vi "Lock VIs.vi"() -> ()   [LabVIEW 2017]
uses:
  KATE/Files/File Utils.lvlib
panel:
  out "Busy":bool
  in  "Reset":bool
  in  "Files":T1(array[cluster]) caption="Folder                                                                                Name                                   Protect"
  in  "Unlock":bool
  in  "Lock":bool
  in  "Get Files":bool
  out "Unlocked Cnt":i32
  out "Locked Cnt":i32
  in  "Lock PW":string="KwestEng#8002"
  in  "Unlock PW":string
  in  "Folder":path
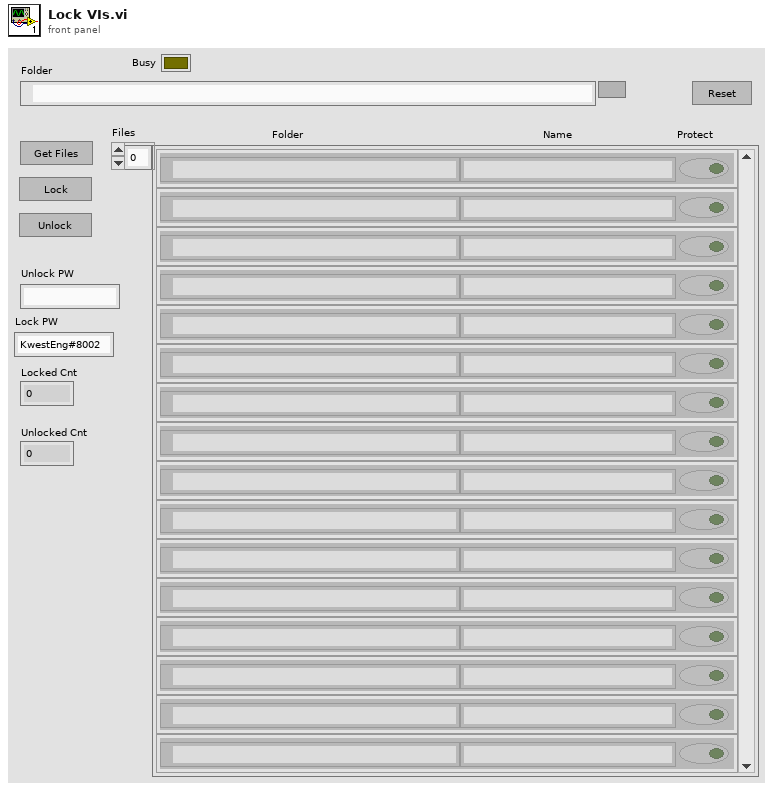
[diagram p1: front panel]
types:
  T1 = cluster{"Name":string, "Folder":path, "Protected":bool}[]
  T2 = cluster{"Name":string, "Folder":path, "Protected":bool}
  T3 = enum32{"invalid lock state", "Not Locked", "Locked (No Password)", "Password-protected"}
  T4 = cluster{"Files":cluster{"Name":string, "Folder":path, "Protected":bool}[], "UnlockPW":string, "LockPW":string}
  T5 = enum8{"Enabled", "Disabled", "Disabled and Grayed Out"}
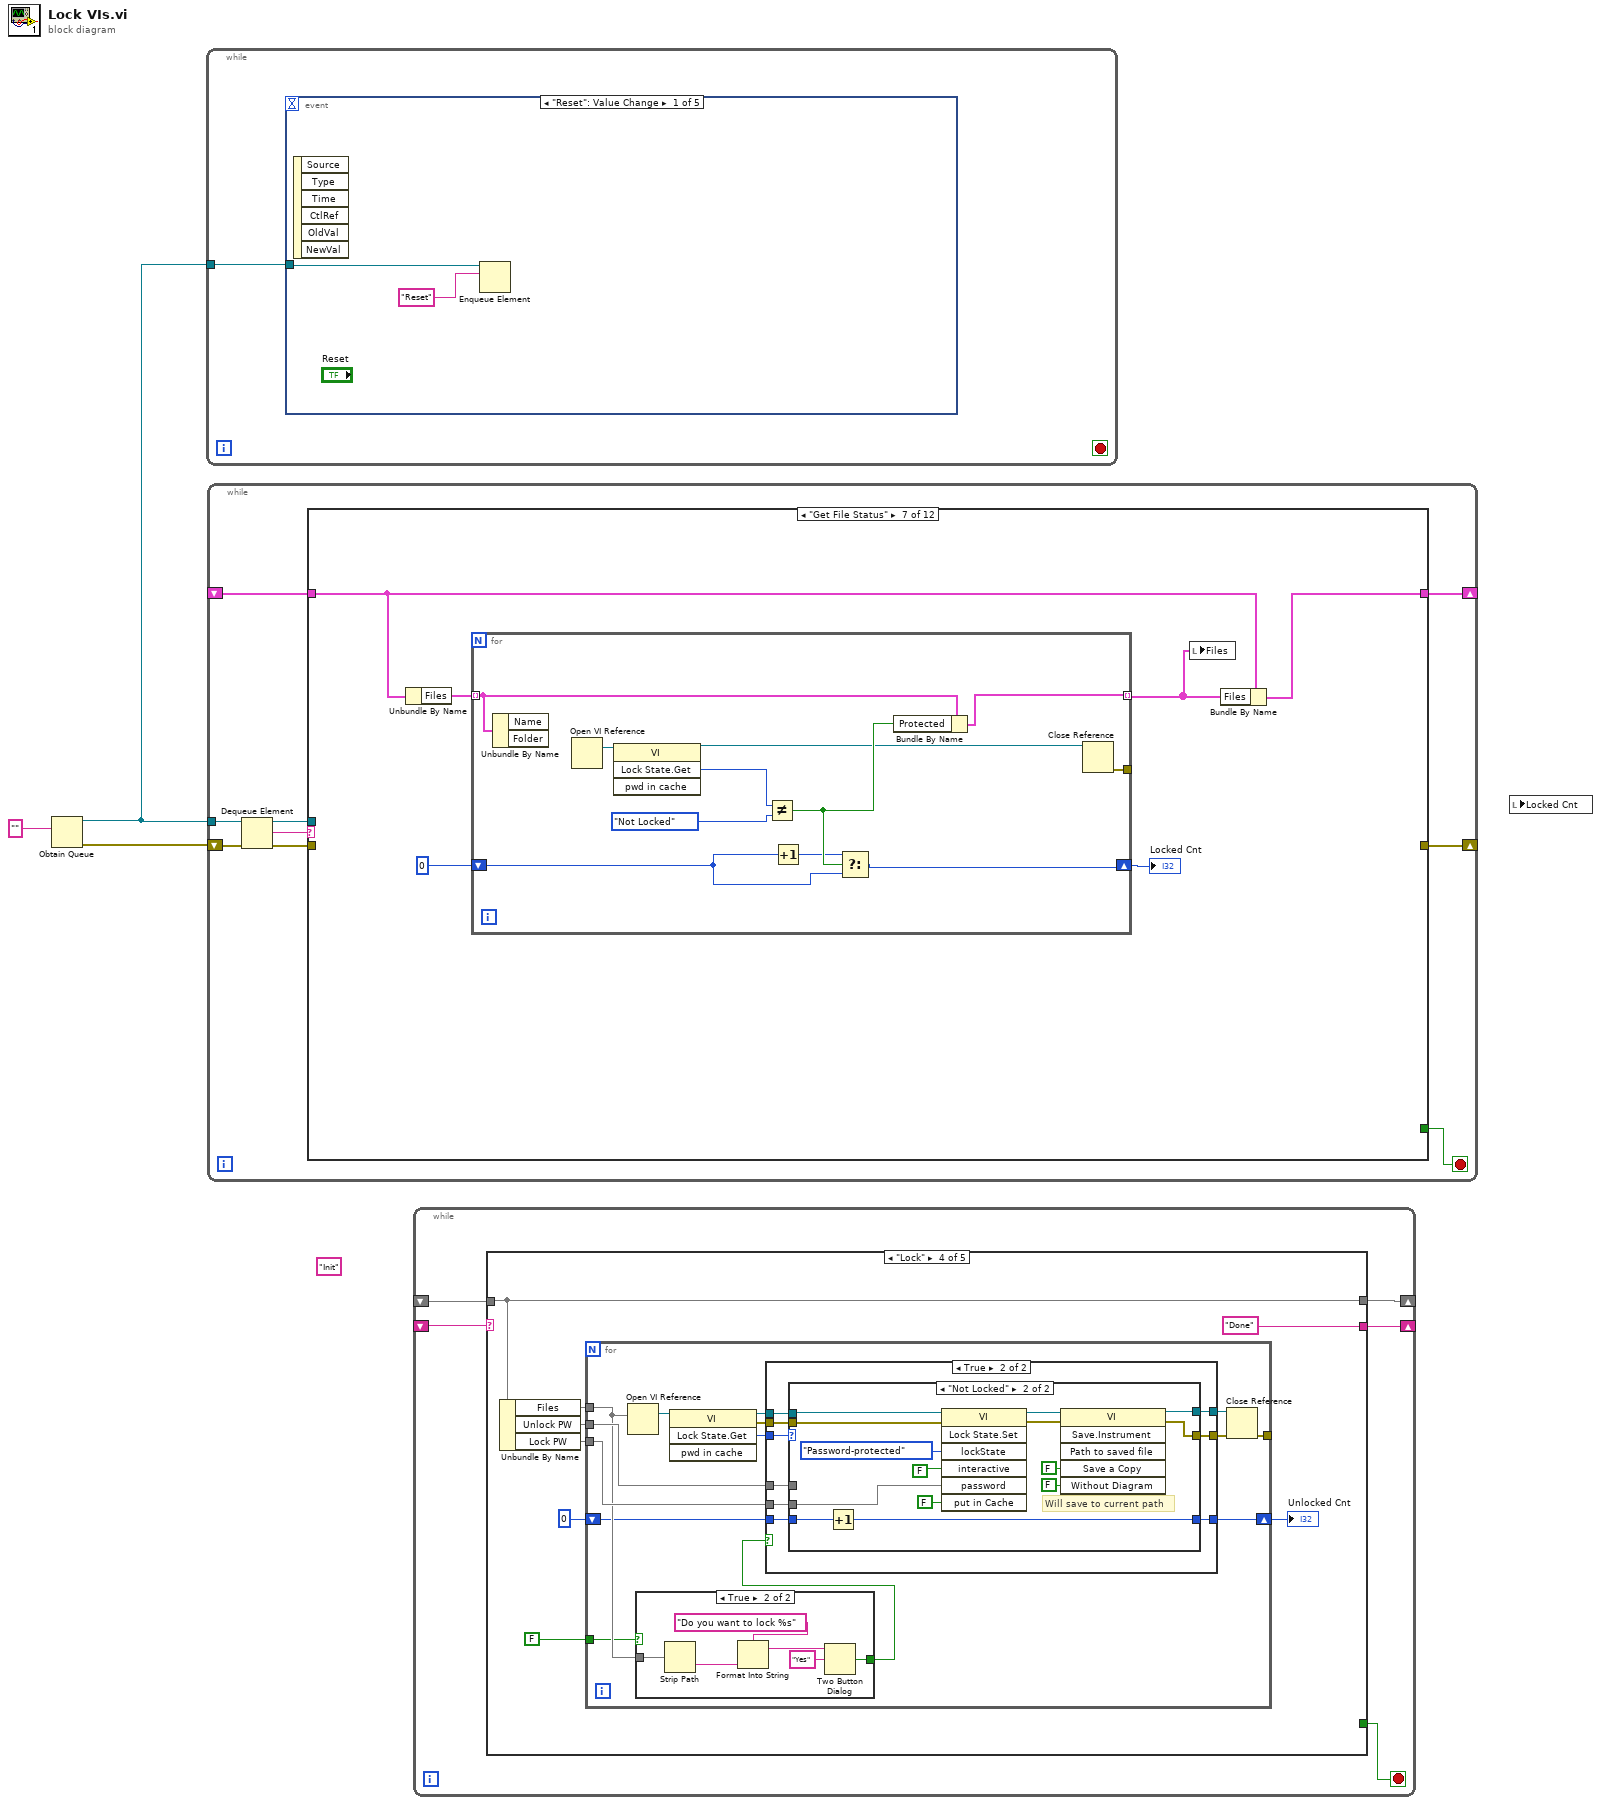
[diagram p0: block diagram]
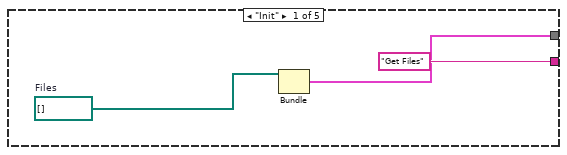
[diagram p2: hidden frame]
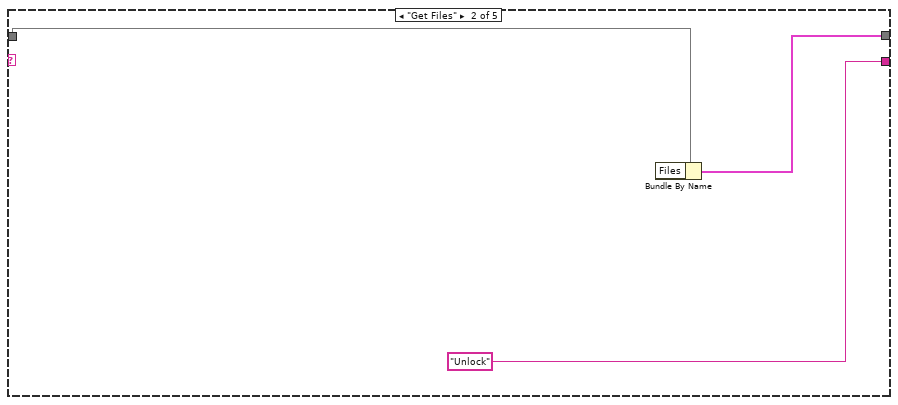
[diagram p3: hidden frame]
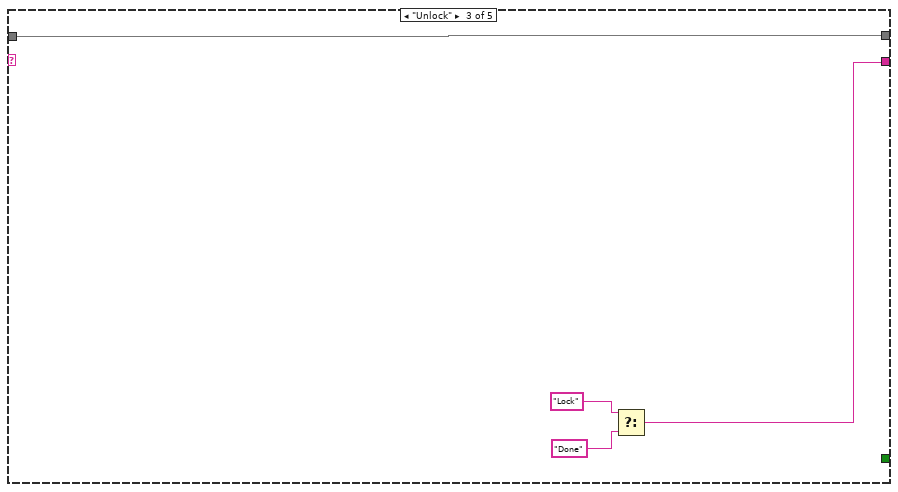
[diagram p4: hidden frame]
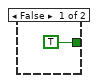
[diagram p5: hidden frame]
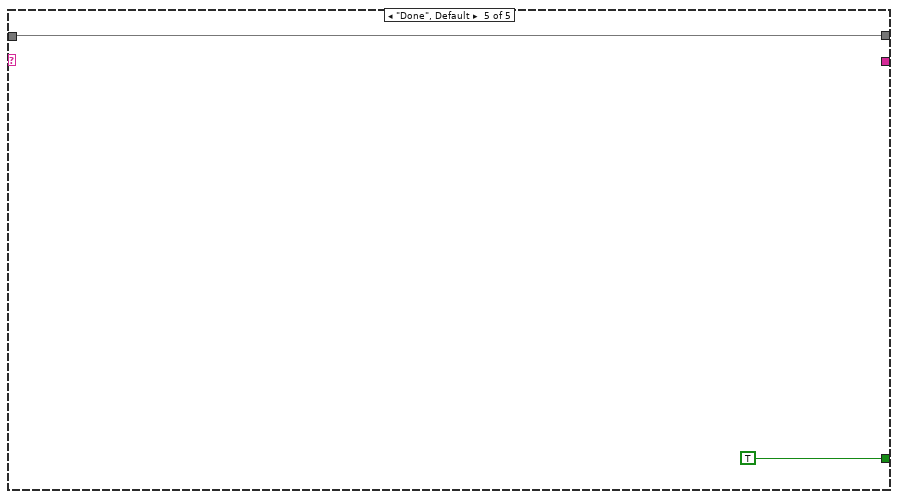
[diagram p8: hidden frame]
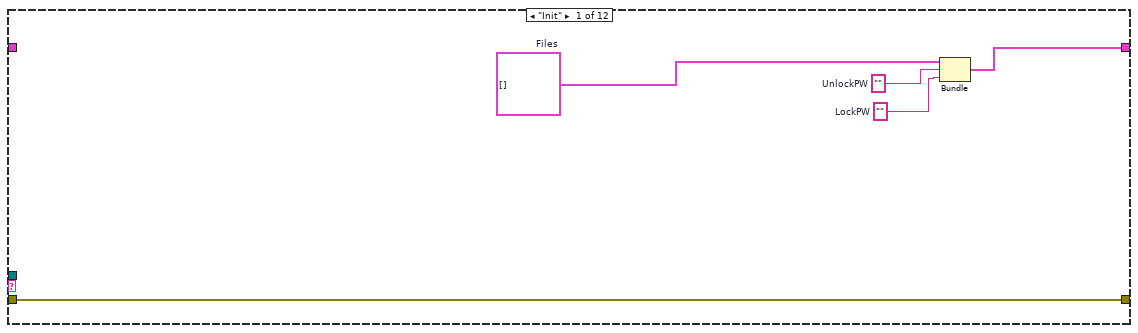
[diagram p9: hidden frame]
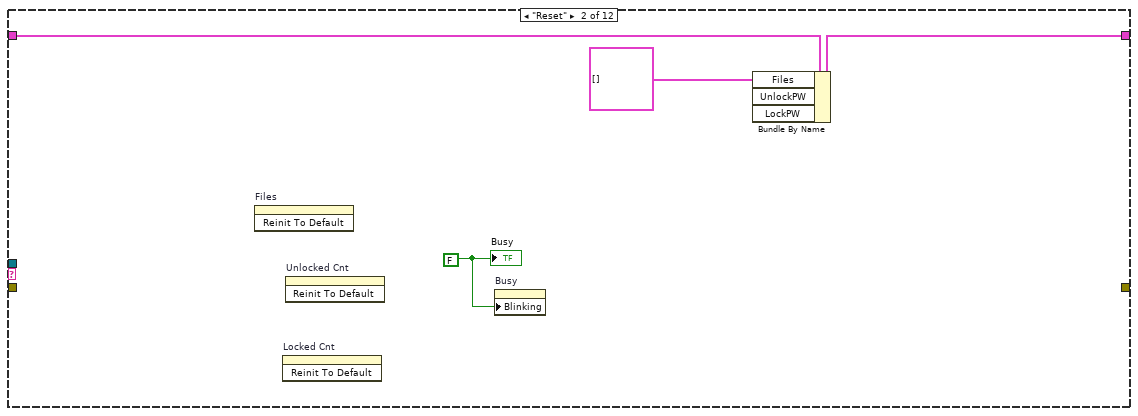
[diagram p10: hidden frame]
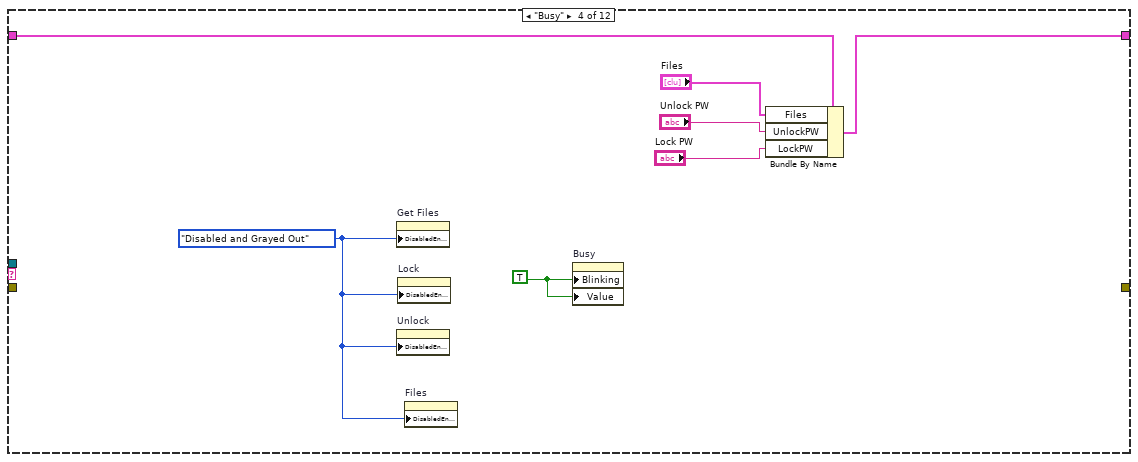
[diagram p12: hidden frame]
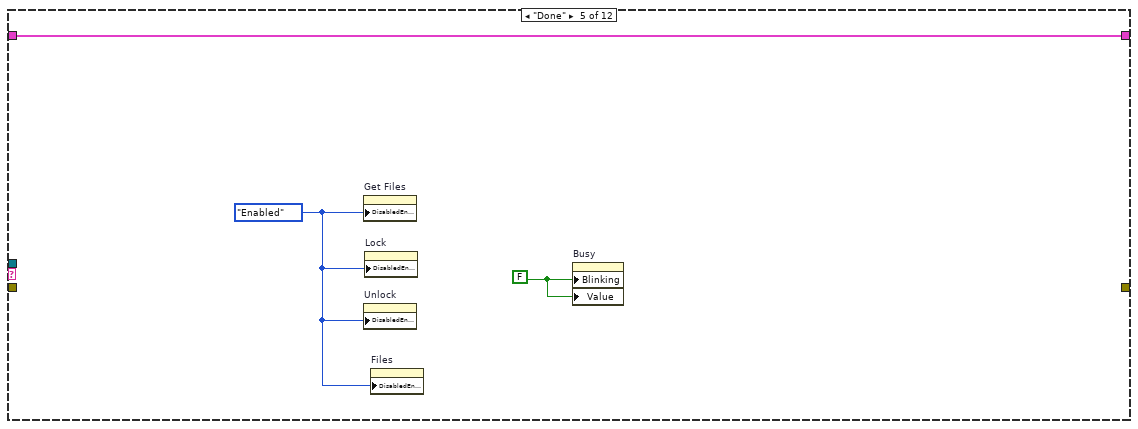
[diagram p13: hidden frame]
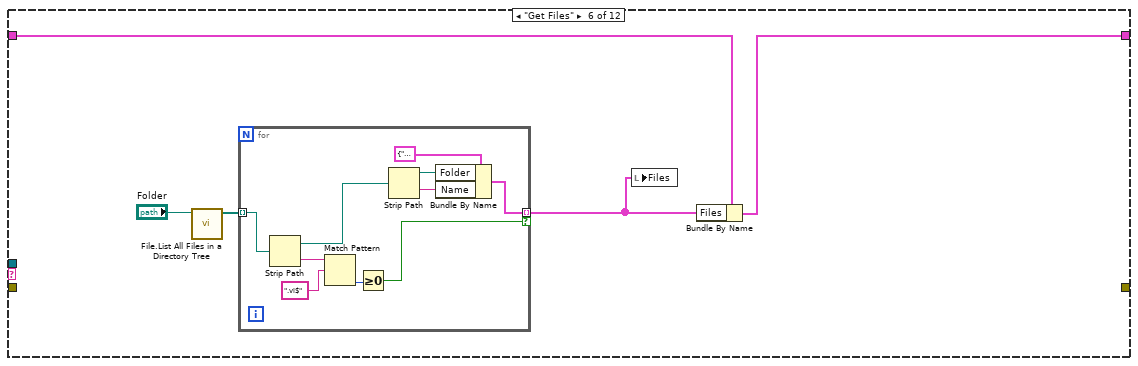
[diagram p14: hidden frame]
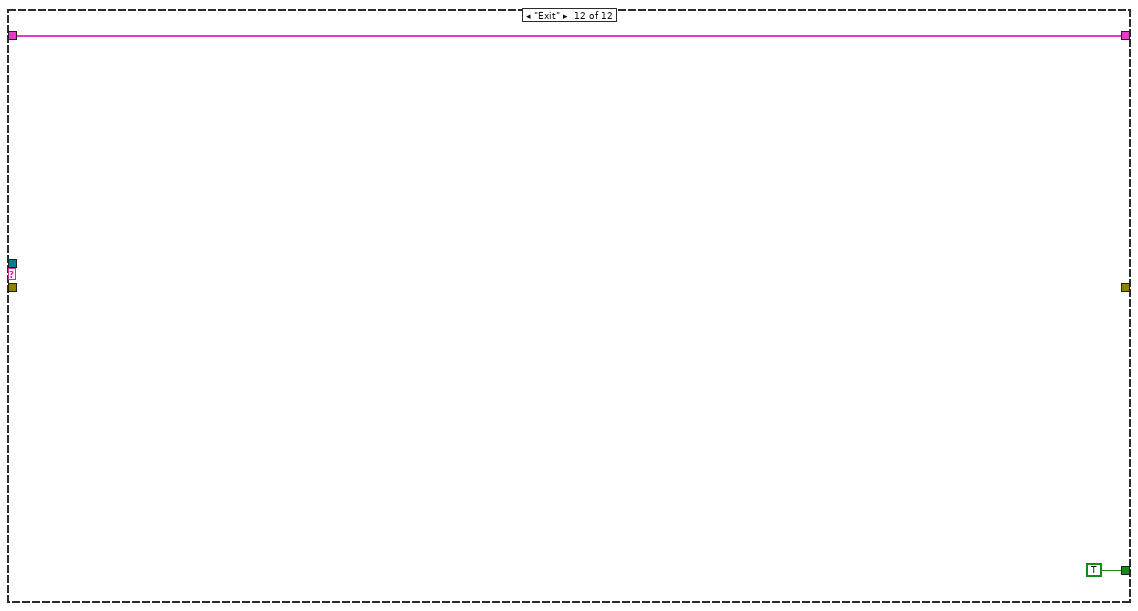
[diagram p19: hidden frame]
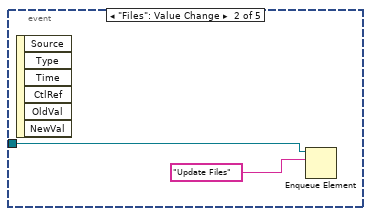
[diagram p20: hidden frame]
diagram:
  (unwired) "Init"
  n1 = Obtain Queue(element data type="") -> (queue out=w3:refnum<queue>, error out=w2:errorcluster)  [unwired: 4 in, 1 out]
  n2 = while {
    tunnel: w3 -> [w5]
    stop <- _ stop-if-true
    n3 = event shown="[0] \"Reset\": Value Change" {
      selector: _ -> [_ _ _ _ _]
      dyn-events: _ -> [_ _ _ _ _]
      timeout: _ -> [_ _ _ _ _]
      tunnel: w5 -> [w7 w8 w11 w15 w19]
      event "Reset": Value Change {
        n4 = event-data() -> ()  [unwired: 1 in, 6 out]
        n5 = Enqueue Element(queue=w7, element="Reset") -> ()  [unwired: 2 in, 3 out]
      }
      event "Files": Value Change {
        n6 = event-data() -> ()  [unwired: 1 in, 6 out]
        n7 = Enqueue Element(queue=w8, element="Update Files") -> ()  [unwired: 2 in, 3 out]
      }
      event "Get Files": Value Change {
        n8 = event-data() -> ()  [unwired: 1 in, 6 out]
        n9 = for {
          tunnel: w11 -> [w13]
          tunnel: string[] ["Busy", "Get Files", "Get File Status", "Done"] -> [w12] mode=indexing
          n10 = Enqueue Element(queue=w13, element=w12) -> ()  [unwired: 2 in, 3 out]
        }
      }
      event "Lock": Value Change {
        n11 = event-data() -> ()  [unwired: 1 in, 6 out]
        n12 = for {
          tunnel: w15 -> [w17]
          tunnel: string[] ["Busy", "Lock", "Done"] -> [w16] mode=indexing
          n13 = Enqueue Element(queue=w17, element=w16) -> ()  [unwired: 2 in, 3 out]
        }
      }
      event "Unlock": Value Change {
        n14 = event-data() -> ()  [unwired: 1 in, 6 out]
        n15 = for {
          tunnel: w19 -> [w21]
          tunnel: string[] ["Busy", "Unlock", "Done"] -> [w20] mode=indexing
          n16 = Enqueue Element(queue=w21, element=w20) -> ()  [unwired: 2 in, 3 out]
        }
      }
    }
  }
  n17 = while {
    tunnel: w3 -> [w29]
    shift-right: [w24] -> _
    shift-left: w2 -> [w26]
    shift-right: [w25] -> _
    shift-left: _ -> [w23]
    stop <- w22 stop-if-true
    n18 = Dequeue Element(queue=w29, error in (no error)=w26) -> (queue out=w30:refnum<queue>, element=w28:string, error out=w27:errorcluster)  [unwired: 1 in, 1 out]
    n19 = case shown="\"Get File Status\"" w28 {
      tunnel: w30 -> [_ _ _ _ _ _ _ _ _ _ _ _]
      tunnel: w27 -> [w32 _ _ _ _ _ _ _ _ _ _ _]
      tunnel: [w34 w37 w40 w43 w50 w52 w67 w83 w84 w85 w86 w88] -> w25
      tunnel: [w32 _ _ _ _ _ _ _ _ _ _ _] -> w24
      tunnel: w23 -> [_ w38 w40 w44 w50 w53 w68 w83 w84 w85 w86 w88]
      tunnel: [_ _ _ _ _ _ _ _ _ _ _ TRUE] -> w22
      frame "Init" {
        w31 = ""  # LockPW
        w33 = ""  # UnlockPW
        w35 = T1 []  # Files
        n20 = Bundle("Files"=w35, "UnlockPW"=w33, "LockPW"=w31) -> (w34:T4)  [unwired: 1 in]
      }
      frame "Reset" {
        w39 = FALSE
        n21 = invoke on="Files" class="Arr (strict)" method="Reinit To Default"() -> ()  [unwired: 3 in, 3 out]
        n22 = invoke on="Locked Cnt" class="DigNum (strict)" method="Reinit To Default"() -> ()  [unwired: 3 in, 3 out]
        n23 = invoke on="Unlocked Cnt" class="DigNum (strict)" method="Reinit To Default"() -> ()  [unwired: 3 in, 3 out]
        n24 = property on="Busy" class="Bool (strict)"("Blinking"=w39) -> ()  [unwired: 2 in, 2 out]
        n25 = Bundle By Name(cluster=w38, "Files"=T1 []) -> (w37:T4)  [unwired: 2 in]
        "Busy" <- w39
      }
      frame "Update Files" {
      }
      frame "Busy" {
        w41 = T5."Disabled and Grayed Out" ("Disabled")
        w47 = TRUE
        n26 = property on="Get Files" class="Bool"("DisabledEnum"=w41) -> ()  [unwired: 2 in, 2 out]
        n27 = property on="Unlock" class="Bool"("DisabledEnum"=w41) -> ()  [unwired: 2 in, 2 out]
        n28 = property on="Lock" class="Bool"("DisabledEnum"=w41) -> ()  [unwired: 2 in, 2 out]
        n29 = property on="Files" class="Arr (strict)"("DisabledEnum"=w41) -> ()  [unwired: 2 in, 2 out]
        n30 = property on="Busy" class="Bool (strict)"("Blinking"=w47, "Value"=w47) -> ()  [unwired: 2 in, 2 out]
        n31 = Bundle By Name(cluster=w44, "Files"="Files", "UnlockPW"="Unlock PW", "LockPW"="Lock PW") -> (w43:T4)
      }
      frame "Done" {
        w48 = T5."Enabled" ("Disabled")
        w49 = FALSE
        n32 = property on="Get Files" class="Bool"("DisabledEnum"=w48) -> ()  [unwired: 2 in, 2 out]
        n33 = property on="Unlock" class="Bool"("DisabledEnum"=w48) -> ()  [unwired: 2 in, 2 out]
        n34 = property on="Lock" class="Bool"("DisabledEnum"=w48) -> ()  [unwired: 2 in, 2 out]
        n35 = property on="Files" class="Arr (strict)"("DisabledEnum"=w48) -> ()  [unwired: 2 in, 2 out]
        n36 = property on="Busy" class="Bool (strict)"("Blinking"=w49, "Value"=w49) -> ()  [unwired: 2 in, 2 out]
      }
      frame "Get Files" {
        n37 = call "File.List All Files in a Directory Tree.vi"("Folder"="Folder") -> ("Files"=w55:path[])  [unwired: 9 in, 1 out]
        n38 = for {
          tunnel: w55 -> [w62] mode=indexing
          tunnel: [w56] -> w51 mode=indexing if=w61
          n39 = Strip Path(path=w62) -> (stripped path=w57:path, name=w65:string)
          n40 = Match Pattern(string=w65, regular expression=".vi$") -> (offset past match=w63:i32)  [unwired: 1 in, 3 out]
          n41 = Greater Or Equal To 0?(x=w63) -> (x >= 0?=w61:bool)
          n42 = Strip Path(path=w57) -> (stripped path=w60:path, name=w58:string)
          n43 = Bundle By Name(cluster=T2 {"Name"="", "Folder"=path "", "Protected"=FALSE} ("File Info"), "Folder"=w60, "Name"=w58) -> (w56:T2)
        }
        n44 = local write "Files"(w51) -> ()
        n45 = Bundle By Name(cluster=w53, "Files"=w51) -> (w52:T4)
      }
      frame "Get File Status" {
        n46 = Unbundle By Name(w68) -> ("Files"=w69:T1)
        n47 = for {
          tunnel: [w81] -> _
          shift-right: [w74] -> w71
          shift-left: 0 -> [w75]
          tunnel: w69 -> [w80] mode=indexing
          tunnel: [w73] -> w66 mode=indexing
          n48 = Unbundle By Name(w80) -> ()  [unwired: 2 out]
          n49 = Open VI Reference() -> (vi reference=w82:refnum<vi>)  [unwired: 6 in, 1 out]
          n50 = invoke class="VI" method="Lock State.Get"(reference=w82) -> (reference out=w72:refnum<vi>, "Get Lock State"=w78:T3)  [unwired: 3 in, 2 out]
          n51 = Not Equal?(x=w78, y=T3."Not Locked" ("Lock State:Get")) -> (x != y?=w77:bool)
          n52 = Increment(x=w75) -> (x+1=w76:i32)
          n53 = Select(t=w76, s=w77, f=w75) -> (s? t:f=w74:i32)
          n54 = Bundle By Name(cluster=w80, "Protected"=w77) -> (w73:T2)
          n55 = Close Reference(reference=w72) -> (error out=w81:errorcluster)  [unwired: 1 in]
        }
        "Locked Cnt" <- w71
        n56 = local write "Files"(w66) -> ()
        n57 = Bundle By Name(cluster=w68, "Files"=w66) -> (w67:T4)
      }
      frame "Unlock" {
      }
      frame "Lock" {
      }
      frame "True" {
      }
      frame "Error", Default {
      }
      frame "Exit" {
      }
    }
  }
  n58 = while {
    shift-right: [w91] -> _
    shift-left: _ -> [w93]
    shift-right: [w92] -> _
    shift-left: [w90] -> w1
    stop <- w89 stop-if-true
    n59 = case shown="\"Lock\"" w90 {
      tunnel: w93 -> [_ w102 w107 w115 w167]
      tunnel: ["Get Files" "Unlock" w103 "Done" _] -> w92
      tunnel: [w96 w101 w107 w115 w167] -> w91
      tunnel: [_ _ _ _ TRUE] -> w89
      frame "Init" {
        w97 = path[] []  # Files
        n60 = Bundle("Files"=w97) -> (w96:cluster{"Files":path[], void, void}, w95, w94)  [unwired: 1 in]
      }
      frame "Get Files" {
        n61 = Bundle By Name(cluster=w102) -> (w101:cluster{}, "Files"=w99:path[])
      }
      frame "Unlock" {
        n62 = Select(t="Lock", f="Done") -> (s=w104:bool, s? t:f=w103:string)
      }
      frame "Lock" {
        n63 = Unbundle By Name(w115) -> ("Files"=w114, "Unlock PW"=w113, "Lock PW"=w112)
        n64 = for {
          tunnel: w114 -> [w120]
          tunnel: w113 -> [w123]
          tunnel: w112 -> [w122]
          tunnel: [w121] -> _
          tunnel: FALSE -> [w118]
          shift-right: [w116] -> w109
          shift-left: 0 -> [w117]
          n65 = Open VI Reference(vi path=w120) -> (vi reference=w129:refnum<vi>)  [unwired: 5 in, 1 out]
          n66 = case shown="True" w118 {
            tunnel: w120 -> [_ w135]
            tunnel: [TRUE w131] -> w119
            frame False {
            }
            frame True {
              n67 = Strip Path(path=w135) -> (name=w134:string)  [unwired: 1 out]
              n68 = Format Into String(format string="Do you want to lock %s" ("message"), w134) -> (resulting string=w133:string)  [unwired: 2 in, 1 out]
              n69 = Two Button Dialog(message=w133, 2:"Yes" ("T button name (\"OK\")")) -> (T button?=w131:bool)  [unwired: 1 in]
            }
          }
          n70 = invoke class="VI" method="Lock State.Get"(reference=w129) -> (reference out=w127:refnum<vi>, error out=w126:errorcluster, "Get Lock State"=w128:T3)  [unwired: 3 in, 1 out]
          n71 = case shown="True" w119 {
            tunnel: w128 -> [_ w148]
            tunnel: w127 -> [w139 w147]
            tunnel: w126 -> [w138 w146]
            tunnel: [w139 w145] -> w125
            tunnel: [w138 w144] -> w124
            tunnel: w123 -> [_ w143]
            tunnel: w122 -> [_ w142]
            tunnel: w117 -> [w137 w141]
            tunnel: [w137 w140] -> w116
            frame False {
            }
            frame True {
              n72 = case shown="\"Not Locked\"" w148 {
                tunnel: w147 -> [w151 w165]
                tunnel: w146 -> [w150 w163]
                tunnel: [w151 w160] -> w145
                tunnel: [w150 w159] -> w144
                tunnel: w143 -> [_ _]
                tunnel: w142 -> [_ w156]
                tunnel: w141 -> [w149 w153]
                tunnel: [w149 w152] -> w140
                frame Default {
                  # "Do Nothing"
                }
                frame "Not Locked" {
                  # "Will save to current path"
                  n73 = Increment(x=w153) -> (x+1=w152:i32)
                  n74 = invoke class="VI" method="Lock State.Set"(reference=w165, error in=w163, "lockState"=T3."Password-protected" ("Lock State"), "interactive"=FALSE ("Put in Cache"), "password"=w156, "put in Cache"=FALSE ("Put in Cache")) -> (reference out=w161:refnum<vi>, error out=w155:errorcluster)  [unwired: 1 in, 5 out]
                  n75 = invoke class="VI" method="Save.Instrument"(reference=w161, error in=w155, "Save a Copy"=FALSE, "Without Diagram"=FALSE) -> (reference out=w160:refnum<vi>, error out=w159:errorcluster)  [unwired: 2 in, 4 out]
                }
              }
            }
          }
          n76 = Close Reference(reference=w125, error in (no error)=w124) -> (error out=w121:errorcluster)
        }
        "Unlocked Cnt" <- w109
      }
      frame "Done", Default {
      }
    }
  }
  n77 = local read "Locked Cnt"() -> ()  [unwired: 1 in]
